vi "Open Private Data Cluster Refs.vi"(8 "error in (no error)":errorcluster, 10 "Calling VI Ref":refnum<vi>, 11 "Application Ref":refnum<vi>) -> (0 "error out":errorcluster, 3 "Private Data Refs":T1)   [LabVIEW 2020, in "Add to Private Data.lvlib"]
uses:
  Add to Private Data.lvlib
  Private Data Refs.ctl
  <vilib>/Utility/error.llb/Error Cluster From Error Code.vi
  <vilib>/ErrorRing/Error Ring.xnode
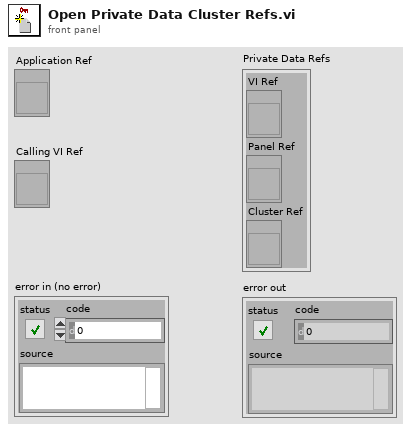
[diagram p1: front panel]
types:
  T1 = typedef "Add to Private Data.lvlib/Private Data Refs.ctl" = cluster{"VI Ref":refnum<vi>, "Panel Ref":refnum<vi>, "Cluster Ref":refnum<vi>}
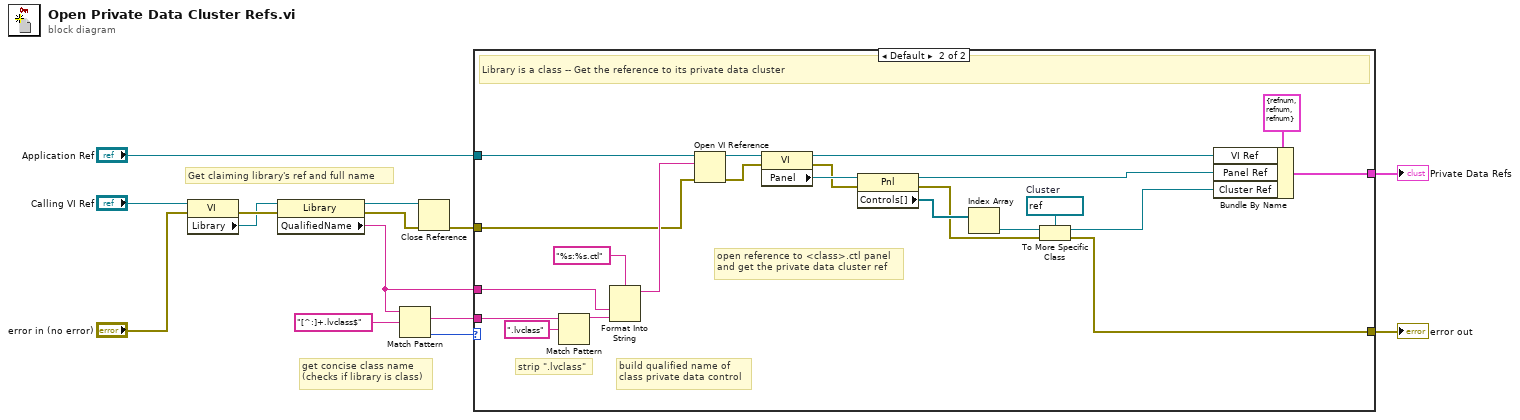
[diagram p0: block diagram]
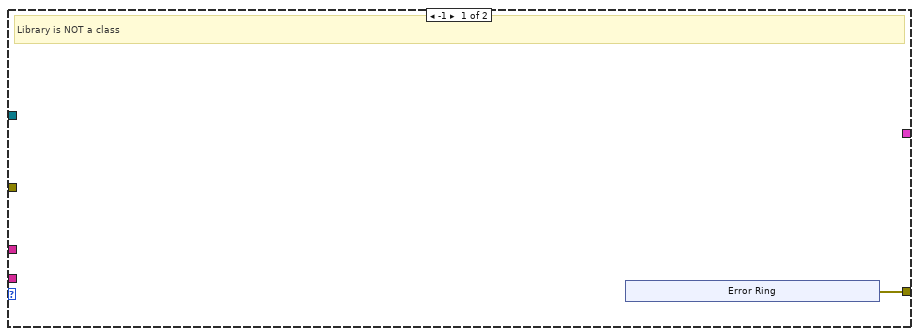
[diagram p2: hidden frame]
diagram:
  # "Get claiming library's ref and full name"
  # "get concise class name\n(checks if library is class)"
  n1 = property on="Property Node" class="VI"(reference="Calling VI Ref", error in="error in (no error)") -> (error out=w6:errorcluster, "Library"=w2:refnum<vi>)  [unwired: 1 out]
  n2 = property on="Property Node" class="Library"(reference=w2, error in=w6) -> (reference out=w7:refnum<vi>, error out=w5:errorcluster, "QualifiedName"=w12:string)
  n3 = Match Pattern(string=w12, regular expression="[^:]+.lvclass$") -> (match substring=w13:string, offset past match=w11:i32)  [unwired: 1 in, 2 out]
  n4 = Close Reference(reference=w7, error in (no error)=w5) -> (error out=w4:errorcluster)
  n5 = case shown="Default" w11 {
    tunnel: w13 -> [_ w35]
    tunnel: w12 -> [_ w36]
    tunnel: "Application Ref" -> [_ w32]
    tunnel: w4 -> [_ w31]
    tunnel: [w15 w26] -> w3
    tunnel: [_ w21] -> w1
    frame -1 {
      # "Library is NOT a class"
      n6 = xnode "Error Ring"() -> ("error out"=w15:errorcluster)
    }
    frame Default {
      w28 = refnum<vi> refnum  # Cluster
      # "open reference to <class>.ctl panel\nand get the private data cluster ref"
      # "build qualified name of\nclass private data control"
      # "strip \".lvclass\""
      # "Library is a class -- Get the reference to its private data cluster"
      n7 = Match Pattern(string=w35, regular expression=".lvclass") -> (before substring=w33:string)  [unwired: 1 in, 3 out]
      n8 = Format Into String(format string="%s:%s.ctl", w36, w33) -> (resulting string=w37:string)  [unwired: 2 in, 1 out]
      n9 = Open VI Reference(application reference (local)=w32, vi path=w37, error in (no error)=w31) -> (vi reference=w42:refnum<vi>, error out=w30:errorcluster)  [unwired: 3 in]
      n10 = property class="VI"(reference=w42, error in=w30) -> (reference out=w25:refnum<vi>, error out=w29:errorcluster, "Panel"=w41:refnum<vi>)
      n11 = property class="Pnl"(reference=w41, error in=w29) -> (reference out=w23:refnum<vi>, error out=w27:errorcluster, "Controls[]"=w40:refnum<vi>[])
      n12 = Index Array(array=w40) -> (element=w39:refnum<vi>)  [unwired: 1 in]
      n13 = To More Specific Class(target class=w28, reference=w39, error in=w27) -> (specific class reference=w22:refnum<vi>, error out=w26:errorcluster)
      n14 = Bundle By Name(cluster=T1 {"VI Ref"=refnum, "Panel Ref"=refnum, "Cluster Ref"=refnum} ("Private Data Refs"), "VI Ref"=w25, "Panel Ref"=w23, "Cluster Ref"=w22) -> (w21:T1)
    }
  }
  "error out" <- w3
  "Private Data Refs" <- w1
